vi "Calculate Velocity and Acceleration.vi"(10 "Loop Runtime (s)":dbl, 11 "Displacement (mm)":dbl) -> (2 "Acceleration (mm/s^2)":dbl, 3 "Velocity (mm/s)":dbl)   [LabVIEW 2017]
panel:
  out "dV":dbl
  out "dS":dbl
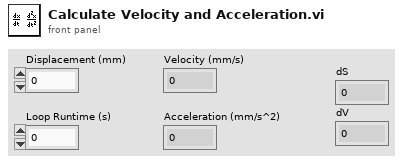
[diagram p1: front panel]
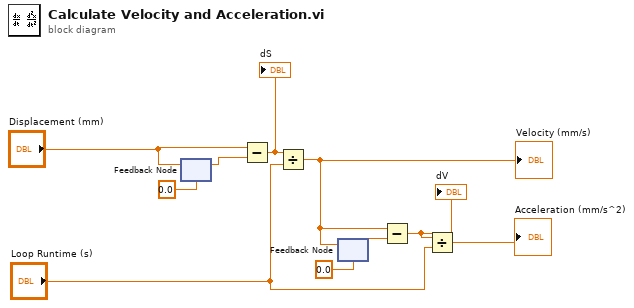
[diagram p0: block diagram]
diagram:
  n1 = feedback #1(0.0 ("Distance (mm)")) -> (w3:dbl)
  n2 = feedback-in #1("Displacement (mm)") -> ()
  n3 = Subtract(x="Displacement (mm)", y=w3) -> (x-y=w4:dbl)
  "dS" <- w4
  n4 = Divide(x=w4, y="Loop Runtime (s)") -> (x/y=w9:dbl)
  "Velocity (mm/s)" <- w9
  n5 = feedback #2(0.0 ("Distance (mm)")) -> (w5:dbl)
  n6 = feedback-in #2(w9) -> ()
  n7 = Subtract(x=w9, y=w5) -> (x-y=w7:dbl)
  "dV" <- w7
  n8 = Divide(x=w7, y="Loop Runtime (s)") -> (x/y=→"Acceleration (mm/s^2)":dbl)
